vi "Detect Threshold.vi"(4 "error in (no error)":errorcluster, 5 "Amplitude":dbl, 7 "Action":T1) -> (0 "error out":errorcluster, 2 "Threshold":dbl)   [LabVIEW 2016]
doc: "The Detect Threshold VI modifies the current value of the threshold based on different events that occur during execution. Use <b>Action</b> to send commands:\n\n<b>Get Threshold</b> to return the current value of the threshold\n<b>Pulse Found</b> which sets the threshold close to the peak that was found\n<b>Pulse Not Found</b> which reduces the threshold to make peaks easier to find"
uses:
  Detect Threshold Control.ctl
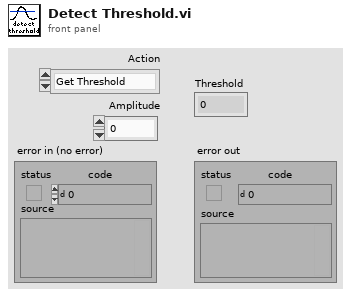
[diagram p1: front panel]
types:
  T1 = typedef "Detect Threshold Control.ctl" = enum16{"Get Threshold", "Pulse Found", "Pulse Not Found"}
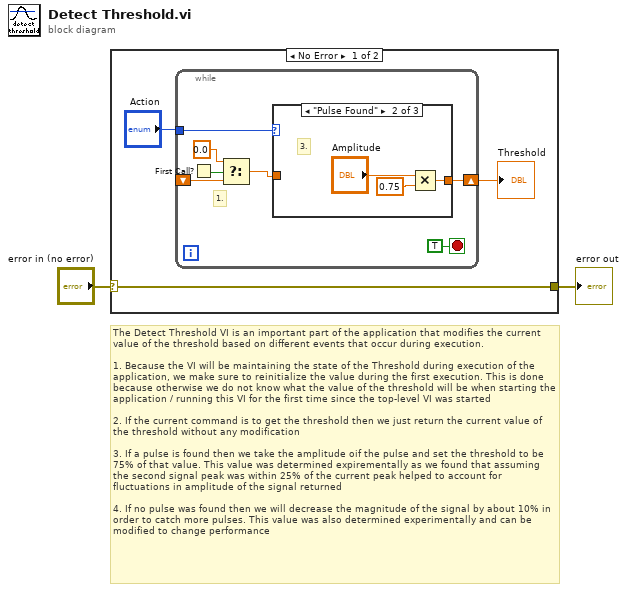
[diagram p0: block diagram]
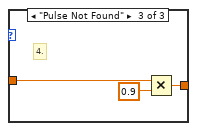
[diagram p3: hidden frame]
diagram:
  # "The Detect Threshold VI is an important part of the application that modifies the current value of the threshold based on different events that occur during execution.\n\n1. Because the VI will be maintaining the state of the Threshold during execution of the application, we make sure to reinitialize the value during the first execution. This is done because otherwise we do not know what the value of the threshold will be when starting the application / running this VI for the first time since the top-level VI was started\n\n2. If the current command is to get the threshold then we just return the current value of the threshold without any modification\n\n3. If a pulse is found then we take the amplitude oif the pulse and set the threshold to be 75% of that value. This value was determined expirementally as we found that assuming the second signal peak was within 25% of the current peak helped to account for fluctuations in amplitude of the signal returned\n\n4. If no pulse was found then we will decrease the magnitude of the signal by about 10% in order to catch more pulses. This value was also determined experimentally and can be modified to change performance"
  n1 = case shown="No Error" "error in (no error)" {
    selector: "error in (no error)" -> [w5 w20]
    tunnel: [w5 w20] -> w1
    frame No Error {
      n2 = while {
        tunnel: "Action" -> [w12]
        shift-right: [w10] -> w4
        shift-left: _ -> [w8]
        stop <- TRUE stop-if-true
        # "1."
        n3 = First Call?() -> (First Call?: T/F=w9:bool)
        n4 = Select(t=0.0 ("element"), s=w9, f=w8) -> (s? t:f=w7:dbl)
        n5 = case shown="\"Pulse Found\"" w12 {
          tunnel: [w13 w14 w17] -> w10
          tunnel: w7 -> [w13 _ w18]
          frame "Get Threshold", Default {
            # "2."
          }
          frame "Pulse Found" {
            # "3."
            n6 = Multiply(x="Amplitude", y=0.75) -> (x*y=w14:dbl)
          }
          frame "Pulse Not Found" {
            # "4."
            n7 = Multiply(x=w18, y=0.9) -> (x*y=w17:dbl)
          }
        }
      }
      "Threshold" <- w4
    }
    frame Error {
    }
  }
  "error out" <- w1
